vi "set_moving_statuses.vi"(8 "error in (no error)":errorcluster caption="错误输入（无错误）", 10 "moving statuses":bool[](array[boolean]), 11 "MotorSystem输入":refnum<class "MotorSystem.lvclass">) -> (0 "error out":errorcluster caption="错误输出", 3 "MotorSystem输出":refnum<class "MotorSystem.lvclass">)   [LabVIEW 2016, in "MotionControl.lvlib" / "MotorSystem.lvclass"]
uses:
  <userlib>/MotionControl/MotorSystem/MotorSystem.lvclass
  <userlib>/MotionControl/MotorSystem/MotorSystem.lvclass/MotorSystem.ctl
  <userlib>/MotionControl/OneMotion/OneMotion.lvclass/OneMotion.ctl
  <userlib>/MotionControl/StepMotor/StepMotor.lvclass/StepMotor.ctl
  <userlib>/MotionControl/StepMotor/StepMotor.lvclass
  <userlib>/MotionControl/OneMotion/OneMotion.lvclass
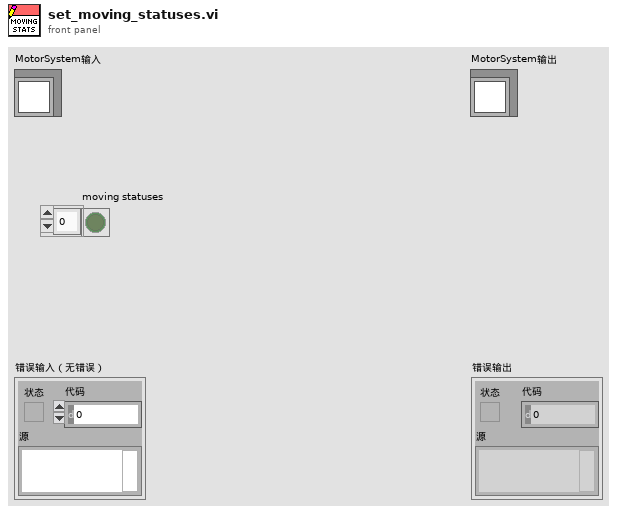
[diagram p1: front panel]
types:
  T1 = typedef "MotionControl.lvlib/MotorSystem.lvclass/MotionCluster.ctl" = cluster{"OneMotion.lvclass":refnum<class "OneMotion.lvclass">, "connected?":bool, "default enabled?":bool, "enabled?":bool}
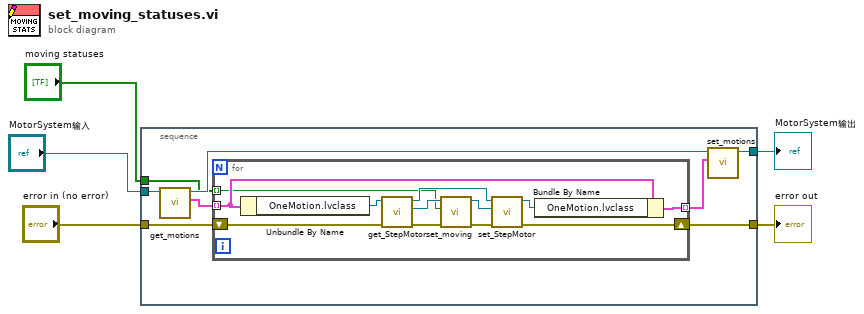
[diagram p0: block diagram]
diagram:
  n1 = stacked-sequence {
    tunnel: [w8] -> w5
    tunnel: [w6] -> w3
    tunnel: "MotorSystem输入" -> [w13]
    tunnel: "error in (no error)" -> [w9]
    tunnel: "moving statuses" -> [w7]
    frame #0 {
      n2 = call <userlib>:"get_motions.vi"("MotorSystem输入"=w13) -> ("motions"=w12:T1[], "MotorSystem输出"=w11:refnum<class "MotorSystem.lvclass">)  [unwired: 8 in, 1 out]
      n3 = for {
        tunnel: w12 -> [w18] mode=indexing
        tunnel: [w17] -> w10 mode=indexing
        shift-right: [w15] -> w8
        shift-left: w9 -> [w16]
        tunnel: w7 -> [w14] mode=indexing
        n4 = Unbundle By Name(w18) -> ("OneMotion.lvclass"=w25:refnum<class "OneMotion.lvclass">)
        n5 = call <userlib>:"get_StepMotor.vi"("error in (no error)"=w16, "OneMotion输入"=w25) -> ("error out"=w20:errorcluster, "StepMotor.lvclass"=w24:refnum<class "StepMotor.lvclass">, "OneMotion输出"=w22:refnum<class "OneMotion.lvclass">)  [unwired: 7 in]
        n6 = call <userlib>:"set_moving.vi"("error in (no error)"=w20, "moving?"=w14, "StepMotor输入"=w24) -> ("error out"=w19:errorcluster, "StepMotor输出"=w23:refnum<class "StepMotor.lvclass">)  [unwired: 7 in]
        n7 = call <userlib>:"set_StepMotor.vi"("error in (no error)"=w19, "StepMotor.lvclass"=w23, "OneMotion输入"=w22) -> ("error out"=w15:errorcluster, "OneMotion输出"=w21:refnum<class "OneMotion.lvclass">)  [unwired: 7 in]
        n8 = Bundle By Name(cluster=w18, "OneMotion.lvclass"=w21) -> (w17:T1)
      }
      n9 = call <userlib>:"set_motions.vi"("motions"=w10, "MotorSystem输入"=w11) -> ("MotorSystem输出"=w6:refnum<class "MotorSystem.lvclass">)  [unwired: 8 in, 1 out]
    }
  }
  "error out" <- w5
  "MotorSystem输出" <- w3
